vi "Configure Voltage.vi"(0 "VISA resource name":refnum<visa-resource-name>, 5 "level (50mV)":u16(ring) items=["50 mV", "100 mV", "250 mV", "500 mV", "1 V", "20 mV"], 7 "offset (0.0V)":u16(ring) items=["0.0 V", "1.5 V", "2.0 V"], 9 "source (0:internal)":u16(ring) items=["internal", "external"], 11 "error in (no error)":errorcluster, 12 "Enable DC Bias Output (enable)":bool=TRUE) -> (4 "VISA resource name out":refnum<visa-resource-name>, 15 "error out":errorcluster)   [LabVIEW 2016, in "Agilent 4263X.lvlib"]
doc: "This VI configures the voltage settings of the instrument."
uses:
  <instrlib>/Agilent 4263X/Agilent 4263X.lvlib
panel:
  # "enable\ndisable"
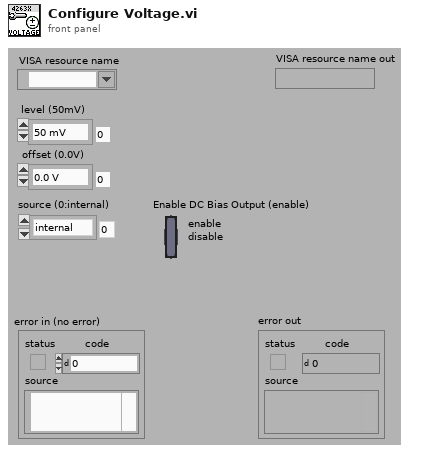
[diagram p1: front panel]
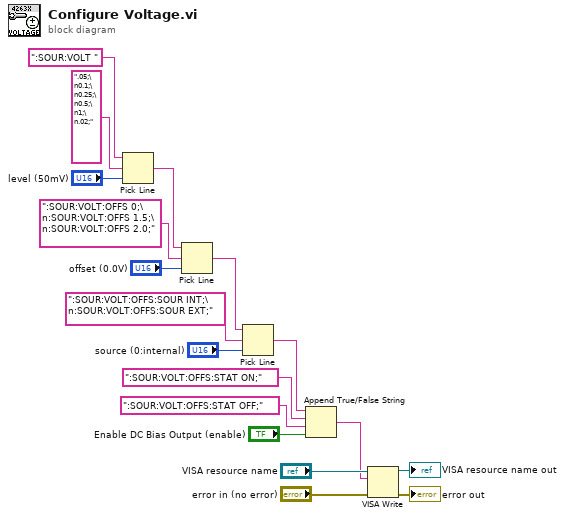
[diagram p0: block diagram]
diagram:
  n1 = Pick Line(string ("")=":SOUR:VOLT ", multi-line string=".05;\n0.1;\n0.25;\n0.5;\n1;\n.02;", line index="level (50mV)") -> (output string=w10:string)
  n2 = Pick Line(string ("")=w10, multi-line string=":SOUR:VOLT:OFFS 0;\n:SOUR:VOLT:OFFS 1.5;\n:SOUR:VOLT:OFFS 2.0;", line index="offset (0.0V)") -> (output string=w1:string)
  n3 = Pick Line(string ("")=w1, multi-line string=":SOUR:VOLT:OFFS:SOUR INT;\n:SOUR:VOLT:OFFS:SOUR EXT;", line index="source (0:internal)") -> (output string=w4:string)
  n4 = Append True/False String(1:"Enable DC Bias Output (enable)", 2:":SOUR:VOLT:OFFS:STAT OFF;", 3:":SOUR:VOLT:OFFS:STAT ON;", 4:w4) -> (0:w2:string)
  n5 = VISA Write(VISA resource name="VISA resource name", write buffer=w2, error in (no error)="error in (no error)") -> (VISA resource name out=→"VISA resource name out":refnum<visa-resource-name>, error out=→"error out":errorcluster)  [unwired: 1 out]
